vi "Cook DAQmxRaw Data.vi"(10 "Cook":bool, 11 "Folder With Raw DAQmx":path) -> ()   [LabVIEW 2017]
doc: "Open a TDMS file with DQAmxRaw data in it, write all of the data to a new file. The DAQmxRaw datatype is used for high throughput data file writing. Raw ADC Data is stored with scaling factors in the DAQmxRaw datatype. The decoding information for this datatype is not provided by NI in the tdms documentation at: http://zone.ni.com/devzone/cda/tut/p/id/5696. This VI demonstrates how a simple VI can be used to open a TDMS file which contains data in the DAQmxRaw data type and write it to another file (this operation converts the data in the file to the supported data types available to users in the TDMS documentation).\n\nThis will convert DAQmx Raw data which is problematic for reading with other tools (http://www.mathworks.com/matlabcentral/fileexchange/44206-converttdms-v10)."
panel:
  out "Error":errorcluster
  in  "Stop":bool
  # "Overview: Very simple utility to read in a TDMS file and the write out data to a new TDMS file (which does not use the DAQmx Raw Data type).\nRequirements: >LabVIEW 2012\nInstructions:\n1. Run the VI.\n2. Select Folder to be converted.\n3. Press OK to Cook button."
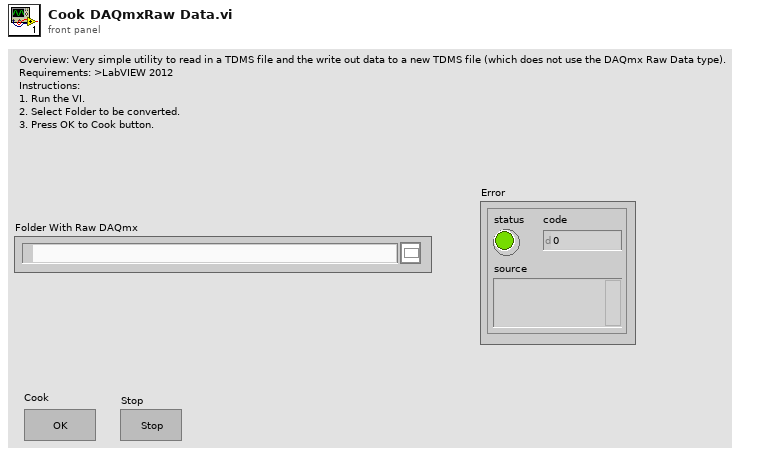
[diagram p1: front panel]
types:
  T1 = enum16{"open", "open or create", "create or replace", "create", "open (read-only)"}
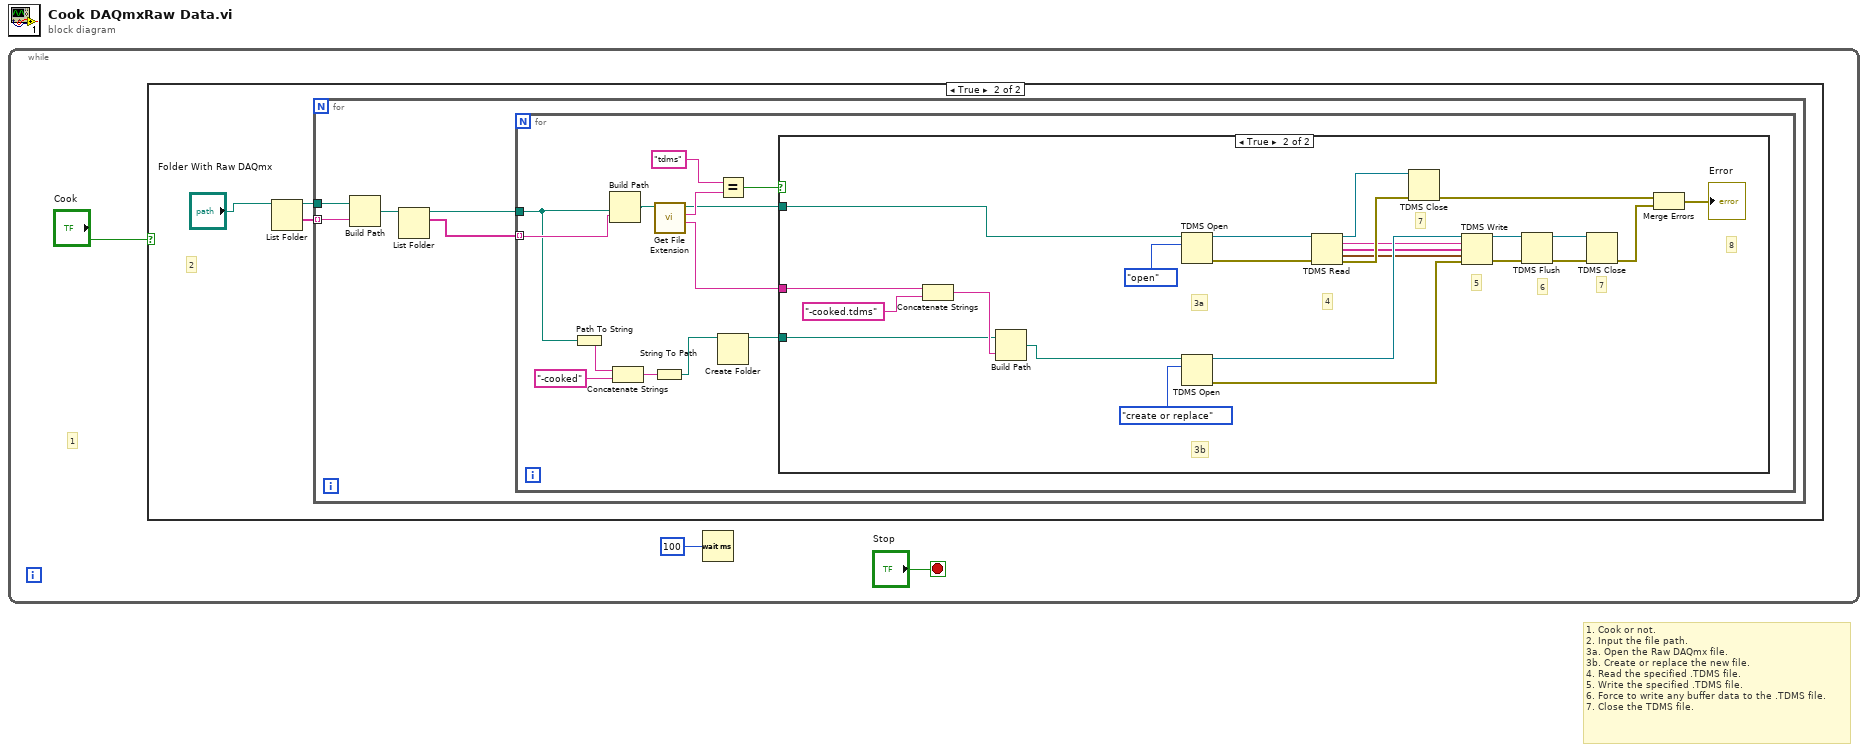
[diagram p0: block diagram]
diagram:
  # "1. Cook or not.\n2. Input the file path.\n3a. Open the Raw DAQmx file.\n3b. Create or replace the new file.\n4. Read the specified .TDMS file.\n5. Write the specified .TDMS file.\n6. Force to write any buffer data to the .TDMS file. \n7. Close the TDMS file."
  n1 = while {
    stop <- "Stop" stop-if-true
    # "1"
    n2 = case shown="True" "Cook" {
      frame False {
      }
      frame True {
        # "2"
        n3 = List Folder(path="Folder With Raw DAQmx") -> (path out=w5:path, folder names=w4:string[])  [unwired: 3 in, 2 out]
        n4 = for {
          tunnel: w5 -> [w9]
          tunnel: w4 -> [w8] mode=indexing
          n5 = Build Path(base path=w9, name or relative path=w8) -> (appended path=w7:path)
          n6 = List Folder(path=w7) -> (path out=w10:path, filenames=w11:string[])  [unwired: 3 in, 2 out]
          n7 = for {
            tunnel: w11 -> [w24] mode=indexing
            tunnel: w10 -> [w17]
            n8 = Path To String(path=w17) -> (string=w16:string)
            n9 = Build Path(base path=w17, name or relative path=w24) -> (appended path=w23:path)
            n10 = Concatenate Strings(w16, "-cooked" ("string")) -> (w14:string)
            n11 = String To Path(string=w14) -> (path=w13:path)
            n12 = call <vilib>:"Get File Extension.vi"("file"=w23) -> ("filename without extension"=w18:string, "lowercase file extension"=w22:string, "dup file"=w19:path)  [unwired: 6 in, 2 out]
            n13 = Equal?(x="tdms", y=w22) -> (x = y?=w20:bool)
            n14 = Create Folder(path (use dialog)=w13) -> (created path=w12:path)  [unwired: 2 in, 2 out]
            n15 = case shown="True" w20 {
              tunnel: w19 -> [_ w30]
              tunnel: w18 -> [_ w28]
              tunnel: w12 -> [_ w25]
              frame False {
              }
              frame True {
                # "3a"
                # "8"
                # "7"
                # "6"
                # "5"
                # "7"
                # "4"
                # "3b"
                n16 = Concatenate Strings(w28, "-cooked.tdms" ("name or relative path")) -> (w26:string)
                n17 = Build Path(base path=w25, name or relative path=w26) -> (appended path=w29:path)
                n18 = TDMS Open(10:T1."open" ("operation (0:open)"), 11:w30) -> (0:w37:errorcluster, 3:w36:refnum<k34>)  [unwired: 5 in]
                n19 = TDMS Open(10:T1."create or replace" ("operation (0:open)"), 11:w29) -> (0:w45:errorcluster, 3:w38:refnum<k34>)  [unwired: 5 in]
                n20 = TDMS Read(0:w36, 11:w37) -> (4:w40:refnum<k34>, 6:w33:string, 8:w34:string[], 10:w35:waveform(dbl)[], 15:w39:errorcluster)  [unwired: 6 in, 1 out]
                n21 = TDMS Close(8:w39, 11:w40) -> (0:w46:errorcluster)  [unwired: 1 out]
                n22 = TDMS Write(0:w38, 5:w33, 7:w34, 9:w35, 11:w45) -> (4:w42:refnum<k34>, 15:w41:errorcluster)  [unwired: 1 in, 2 out]
                n23 = TDMS Flush(4:w41, 7:w42) -> (0:w43:errorcluster, 3:w44:refnum<k34>)
                n24 = TDMS Close(8:w43, 11:w44) -> (0:w47:errorcluster)  [unwired: 1 out]
                n25 = Merge Errors(w46, w47) -> (→"Error":errorcluster)
              }
            }
          }
        }
      }
    }
    n26 = Wait (ms)(milliseconds to wait=u32 100 ("millisecond multiple")) -> ()  [unwired: 1 out]
  }
